vi "Close refnum.vi"(1 "Data IN":T1 caption="Data") -> (0 "Data OUT":T1 caption="Data")   [LabVIEW 2013]
uses:
  PDF Table Data.ctl
  C:/Users/MaxCorp/Documents/GitHub/TopView/DLL/itextsharp.dll
  DLL/itextsharp.dll
  PDF Table XControl.xctl
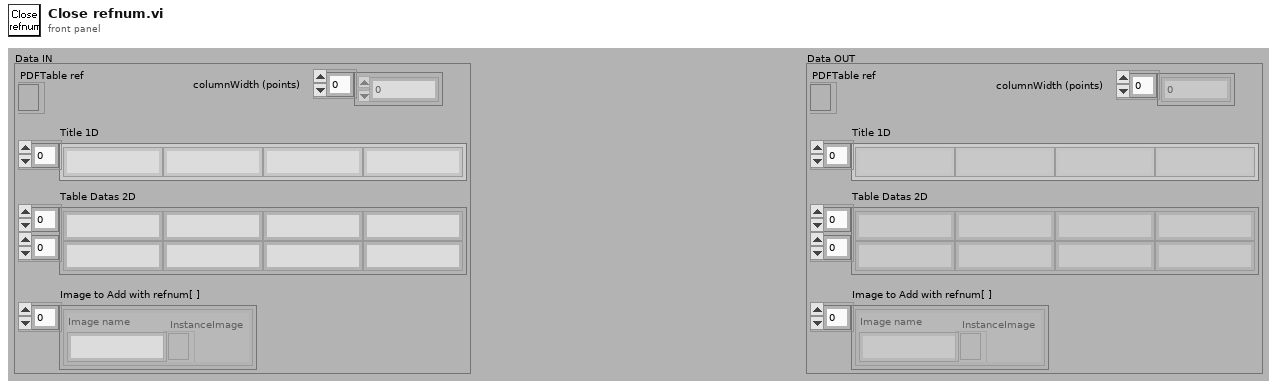
[diagram p1: front panel]
types:
  T1 = typedef "PDF Table XControl.xctl/PDF Table Data.ctl" = cluster{"PDFTable ref":refnum<k24>, "columnWidth (points)":sgl[], "Title 1D":string[], "Table Datas 2D":string[][], "Image to Add with refnum[ ]":cluster{"Image name":string, "InstanceImage":refnum<k24>}[]}
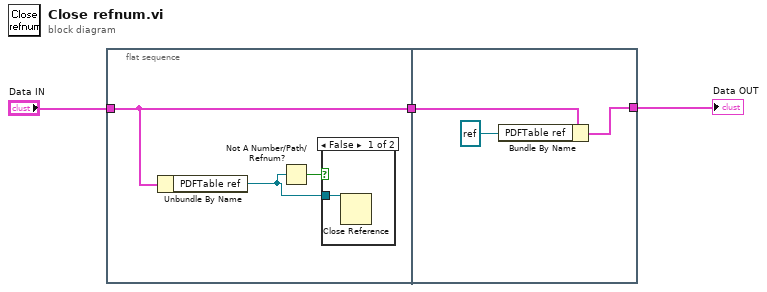
[diagram p0: block diagram]
diagram:
  n1 = flat-sequence {
    tunnel: "Data IN" -> [w4]
    tunnel: [w4] -> w2
    tunnel: w2 -> [w9]
    tunnel: [w8] -> w1
    frame #0 {
      n2 = Unbundle By Name(w4) -> ("PDFTable ref"=w5:refnum<k24>)
      n3 = Not A Number/Path/Refnum?(number/path/refnum=w5) -> (NaN/Path/Refnum?=w6:bool)
      n4 = case shown="False" w6 {
        tunnel: w5 -> [w7 _]
        frame False {
          n5 = Close Reference(reference=w7) -> ()  [unwired: 1 in, 1 out]
        }
        frame True {
        }
      }
    }
    frame #1 {
      n6 = Bundle By Name(cluster=w9, "PDFTable ref"=refnum<k24> refnum) -> (w8:T1)
    }
  }
  "Data OUT" <- w1
